vi "List columns.vi"(8 "error in (no error)":errorcluster, 9 "显示关键参数":bool, 10 "table":string, 11 "database":string="database1.mdb") -> (0 "error out":errorcluster, 3 "columns":string[](array[string]))   [LabVIEW 2016, in "数据查询.lvlib"]
uses:
  <vilib>/addons/database/Connection.llb/DB Tools Open Connec (String).vi
  <userlib>/_LVST/sqlite_api/Core/Tables/SQLite_List Columns.vi
  <userlib>/_OpenG.lib/array/array.llb/Filter 1D Array (String)__ogtk.vi
  <vilib>/addons/database/NI_Database_API.lvlib
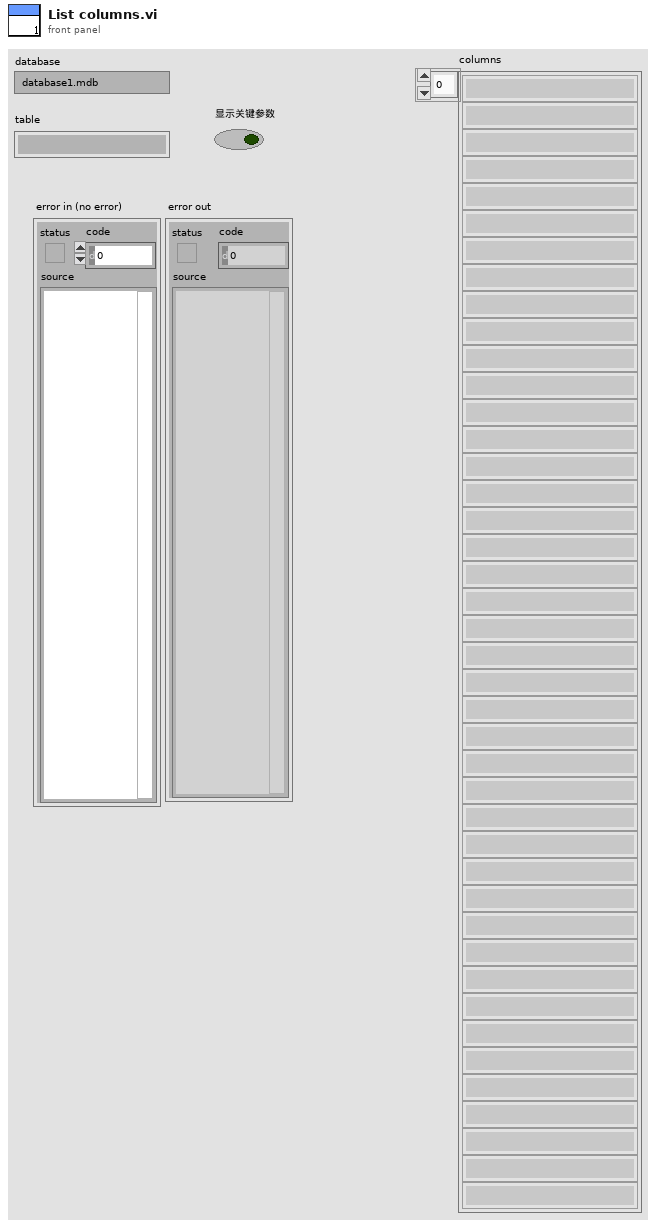
[diagram p1: front panel]
types:
  T1 = typedef "数据库类型.ctl" = enum16{"Access", "SQLite"}
  T2 = typedef "NI_Database_API.lvlib/Conn ObjectReference.ctl" = refnum<k1>
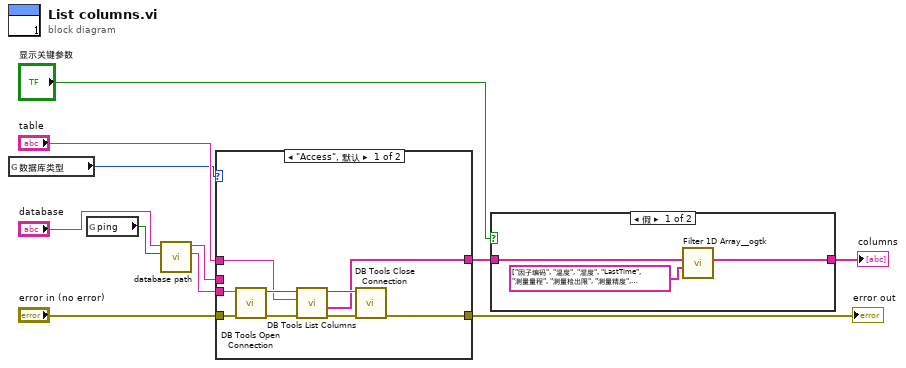
[diagram p0: block diagram]
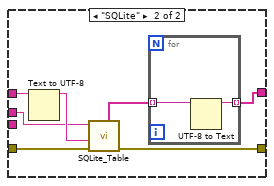
[diagram p3: hidden frame]
diagram:
  n1 = global read "外部调用接口全局变量.vi" "数据库类型"() -> (w1:T1)
  n2 = global read "全局变量.vi" "ping"() -> (w6:bool)
  n3 = call "database path.vi"("ping"=w6, "database"="database") -> ("Connection information"=w2:string, "Path out"=w7:string)  [unwired: 8 in]
  n4 = case shown="\"Access\", 默认" w1 {
    tunnel: "table" -> [w16 w23]
    tunnel: "error in (no error)" -> [w15 w26]
    tunnel: [w14 w27] -> w9
    tunnel: [w13 w24] -> w4
    tunnel: w7 -> [_ w21]
    tunnel: w2 -> [w12 _]
    frame "Access", Default {
      n5 = call-poly <vilib>:"DB Tools Open Connection.vi"("error in (no error)"=w15, "connection information"=w12) -> ("error out"=w18:errorcluster, "connection reference"=w20:T2)  [unwired: 6 in]
      n6 = call <vilib>:"DB Tools List Columns.vi"("error in (no error)"=w18, "table"=w16, "connection reference"=w20) -> ("error out"=w17:errorcluster, "columns"=w13:string[], "connection reference out"=w19:T2)  [unwired: 1 in, 1 out]
      n7 = call <vilib>:"DB Tools Close Connection.vi"("error in (no error)"=w17, "connection reference"=w19) -> ("error out"=w14:errorcluster)  [unwired: 5 in]
    }
    frame "SQLite" {
      n8 = Text to UTF-8(11:w23) -> (3:w22:string)  [unwired: 2 in, 1 out]
      n9 = call-poly <userlib>:"SQLite_Table.vi"("DB Path"=w21, "Table Name"=w22, "error in (no error)"=w26) -> ("Columns"=w25:string[], "error out"=w27:errorcluster)  [unwired: 4 in, 2 out]
      n10 = for {
        tunnel: w25 -> [w29] mode=indexing
        tunnel: [w28] -> w24 mode=indexing
        n11 = UTF-8 to Text(11:w29) -> (3:w28:string)  [unwired: 2 in, 1 out]
      }
    }
  }
  "error out" <- w9
  n12 = case shown="假" "显示关键参数" {
    tunnel: w4 -> [w32 w33]
    tunnel: [w30 w33] -> w3
    frame False {
      n13 = call-poly <userlib>:"Filter 1D Array__ogtk.vi"("items to filter"=string[] ["因子编码", "温度", "湿度", "LastTime", "测量量程", "测量检出限", "测量精度", "测量间隔", "消解温度", "消解时长", "三项式系数", "二次多项式系数", "曲线斜率", "曲线截距", "线性相关系数", "空白校准时间", "标样校准时间", "测量信号值", "稀释倍数", "空白标定系数", "量程系数", "X1"] ("columns"), "array"=w32) -> ("filtered array"=w30:string[])  [unwired: 4 in, 1 out]
    }
    frame True {
    }
  }
  "columns" <- w3
